vi "RotationRoundOff.vi"(7 "Rot IN":dbl) -> (8 "Rounded Rot":dbl)   [LabVIEW 2011]
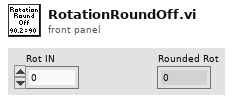
[diagram p1: front panel]
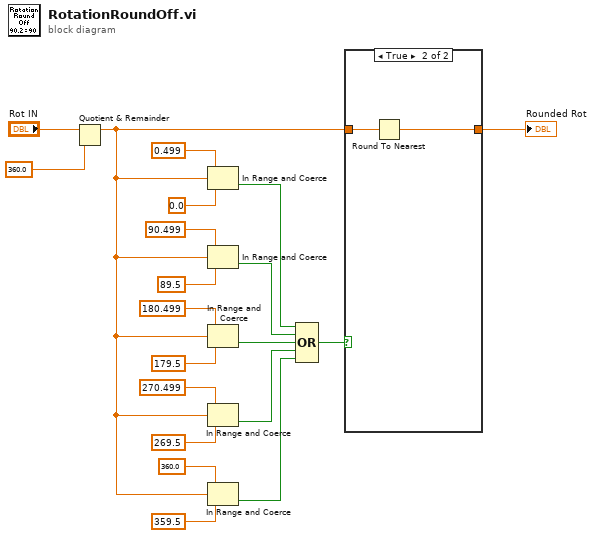
[diagram p0: block diagram]
diagram:
  n1 = Quotient & Remainder(x="Rot IN", y=360.0) -> (x-y*floor(x/y)=w6:dbl)  [unwired: 1 out]
  n2 = In Range and Coerce(upper limit=0.499, x=w6, lower limit=0.0) -> (In Range?=w11:bool)  [unwired: 1 out]
  n3 = In Range and Coerce(upper limit=90.499, x=w6, lower limit=89.5 ("upper limit")) -> (In Range?=w10:bool)  [unwired: 1 out]
  n4 = In Range and Coerce(upper limit=180.499, x=w6, lower limit=179.5 ("upper limit")) -> (In Range?=w9:bool)  [unwired: 1 out]
  n5 = In Range and Coerce(upper limit=270.499, x=w6, lower limit=269.5 ("upper limit")) -> (In Range?=w8:bool)  [unwired: 1 out]
  n6 = In Range and Coerce(upper limit=360.0 ("lower limit"), x=w6, lower limit=359.5 ("upper limit")) -> (In Range?=w7:bool)  [unwired: 1 out]
  n7 = Compound Arithmetic op=OR(w11, w10, w9, w8, w7) -> (w12:bool)
  n8 = case shown="True" w12 {
    tunnel: w6 -> [w21 w23]
    tunnel: [w21 w22] -> w5
    frame False {
    }
    frame True {
      n9 = Round To Nearest(number=w23) -> (nearest integer value=w22:dbl)
    }
  }
  "Rounded Rot" <- w5
